vi "MP Test Path.vi"   [LabVIEW 2019]
uses:
  <vilib>/Rock Robotics/WPI/ThirdParty/Phoenix-LabVIEW/Motor Controller/Controls/CTRE_Phoenix_MotorControl_MotionProfileTrajectoryPoint.ctl
  <vilib>/Utility/file.llb/Read Delimited Spreadsheet (string).vi
  <vilib>/Rock Robotics/WPI/ThirdParty/Phoenix-LabVIEW/Motor Controller/Closed Loop/Motion Profile/CTRE_Phoenix_MotorControl_BufferedTrajectoryPointStream_WriteAll.vi
types:
  T1 = typedef "CTRE_Phoenix_MotorControl_MotionProfileTrajectoryPoint.ctl" = cluster{"Position":dbl, "Velocity":dbl, "Arbitrary Feed Forward":dbl, "Auxiliary Position":dbl, "Auxiliary Velocity":dbl, "Auxiliary Arbitrary Feed Forward":dbl, "Profile Slot Select":i32, "Auxiliary Profile Slot Select":i32, "isLastPoint?":bool, "Zero Position?":bool, "durationMs":u32, "Use Aux PID?":bool}
  T2 = typedef "CTRE_Phoenix_MotorControl_BufferedTrajectoryPointStream_DeviceRef.ctl" = cluster{"Handle":u64, "Library Path":path}
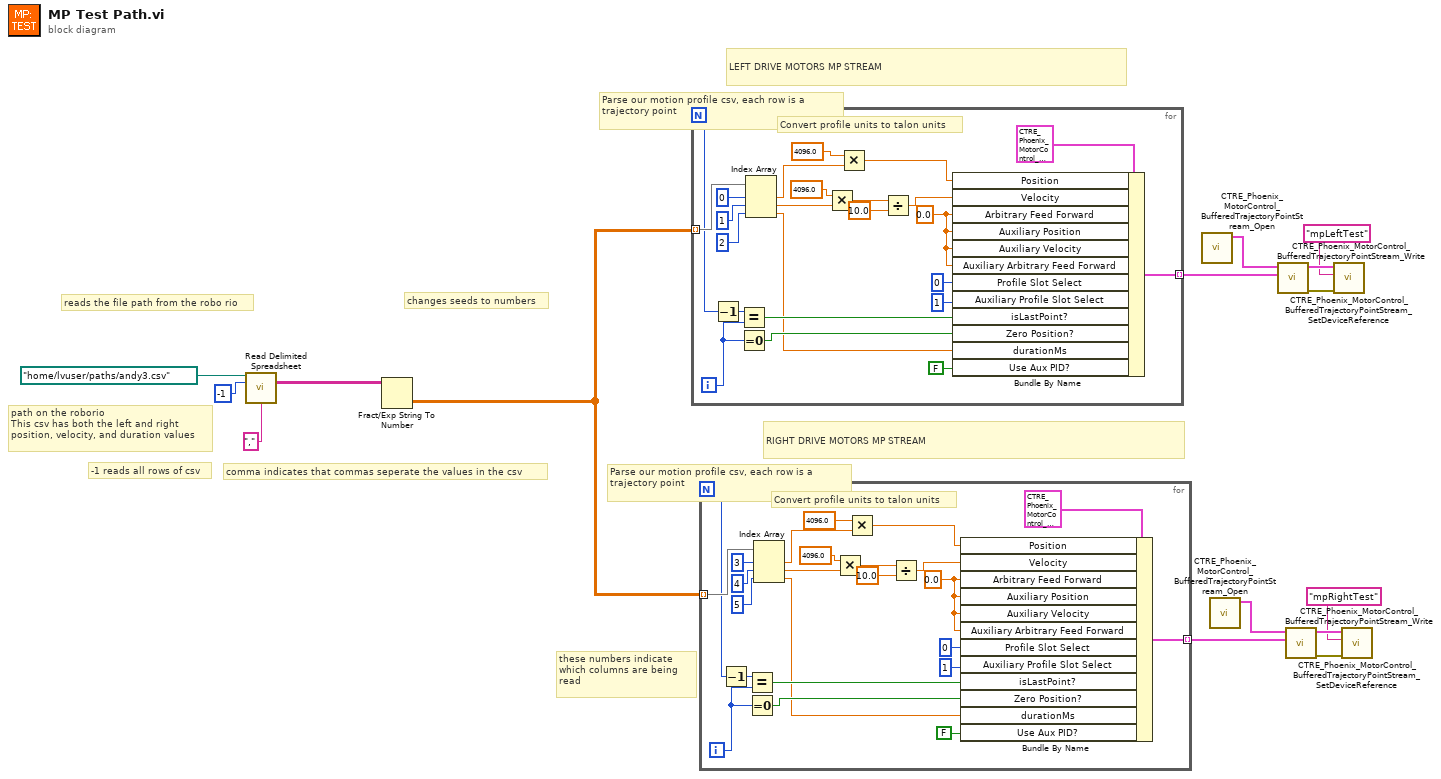
[diagram p0: block diagram]
diagram:
  # "these numbers indicate \nwhich columns are being \nread"
  # "Parse our motion profile csv, each row is a trajectory point"
  # "LEFT DRIVE MOTORS MP STREAM"
  # "Parse our motion profile csv, each row is a trajectory point"
  # "path on the roborio\nThis csv has both the left and right\nposition, velocity, and duration values"
  # "changes seeds to numbers"
  # "comma indicates that commas seperate the values in the csv"
  # "-1 reads all rows of csv"
  # "reads the file path from the robo rio"
  # "RIGHT DRIVE MOTORS MP STREAM"
  n1 = call-poly <vilib>:"Read Delimited Spreadsheet.vi"("file path (dialog if empty)"=path "/home/lvuser/paths/andy3.csv" ("file path (use dialog)"), "number of rows (all:-1)"=-1, "delimiter (\\t)"="," ("delimiter (\\t)")) -> ("all rows"=w1:string[][])  [unwired: 7 in, 5 out]
  n2 = Fract/Exp String To Number(string=w1) -> (number=w2:dbl[][])  [unwired: 3 in, 1 out]
  n3 = for {
    N -> [w32]
    tunnel: w2 -> [w38] mode=indexing
    tunnel: [w28] -> w3 mode=indexing
    i -> [w31]
    w37 = 0.0 ("Arbitrary Feed Forward")
    # "Convert profile units to talon units"
    n4 = Decrement(x=w32) -> (x-1=w33:i32)
    n5 = Equal?(x=w33, y=w31) -> (x = y?=w34:bool)
    n6 = Equal To 0?(x=w31) -> (x = 0?=w30:bool)
    n7 = Index Array(array=w38, index #1=0 ("index"), index #2=1 ("index"), index #3=2 ("index")) -> (element #1=w26:dbl, element #2=w20:dbl, element #3=w27:dbl)
    n8 = Multiply(x=4096.0, y=w20) -> (x*y=w22:dbl)
    n9 = Multiply(x=4096.0, y=w26) -> (x*y=w24:dbl)
    n10 = Divide(x=w22, y=10.0) -> (x/y=w19:dbl)
    n11 = Bundle By Name(cluster=T1 {"Position"=0.0, "Velocity"=0.0, "Arbitrary Feed Forward"=0.0, "Auxiliary Position"=0.0, "Auxiliary Velocity"=0.0, "Auxiliary Arbitrary Feed Forward"=0.0, "Profile Slot Select"=0, "Auxiliary Profile Slot Select"=0, "isLastPoint?"=FALSE, "Zero Position?"=FALSE, "durationMs"=0, "Use Aux PID?"=FALSE} ("Trajectory Point"), "Position"=w24, "Velocity"=w19, "Arbitrary Feed Forward"=w37, "Auxiliary Position"=w37, "Auxiliary Velocity"=w37, "Auxiliary Arbitrary Feed Forward"=w37, "Profile Slot Select"=0, "Auxiliary Profile Slot Select"=1, "isLastPoint?"=w34, "Zero Position?"=w30, "durationMs"=w27, "Use Aux PID?"=FALSE) -> (w28:T1)
  }
  n12 = for {
    N -> [w56]
    tunnel: w2 -> [w62] mode=indexing
    tunnel: [w52] -> w11 mode=indexing
    i -> [w55]
    w61 = 0.0 ("Arbitrary Feed Forward")
    # "Convert profile units to talon units"
    n13 = Decrement(x=w56) -> (x-1=w57:i32)
    n14 = Equal?(x=w57, y=w55) -> (x = y?=w58:bool)
    n15 = Equal To 0?(x=w55) -> (x = 0?=w54:bool)
    n16 = Index Array(array=w62, index #1=3 ("index"), index #2=4 ("index"), index #3=5 ("index")) -> (element #1=w50:dbl, element #2=w44:dbl, element #3=w51:dbl)
    n17 = Multiply(x=4096.0, y=w44) -> (x*y=w46:dbl)
    n18 = Multiply(x=4096.0, y=w50) -> (x*y=w48:dbl)
    n19 = Divide(x=w46, y=10.0) -> (x/y=w43:dbl)
    n20 = Bundle By Name(cluster=T1 {"Position"=0.0, "Velocity"=0.0, "Arbitrary Feed Forward"=0.0, "Auxiliary Position"=0.0, "Auxiliary Velocity"=0.0, "Auxiliary Arbitrary Feed Forward"=0.0, "Profile Slot Select"=0, "Auxiliary Profile Slot Select"=0, "isLastPoint?"=FALSE, "Zero Position?"=FALSE, "durationMs"=0, "Use Aux PID?"=FALSE} ("Trajectory Point"), "Position"=w48, "Velocity"=w43, "Arbitrary Feed Forward"=w61, "Auxiliary Position"=w61, "Auxiliary Velocity"=w61, "Auxiliary Arbitrary Feed Forward"=w61, "Profile Slot Select"=0, "Auxiliary Profile Slot Select"=1, "isLastPoint?"=w58, "Zero Position?"=w54, "durationMs"=w51, "Use Aux PID?"=FALSE) -> (w52:T1)
  }
  n21 = call <vilib>:"CTRE_Phoenix_MotorControl_BufferedTrajectoryPointStream_Open.vi"() -> ("BufferedTrajectoryPointStream_DevRef"=w15:T2)  [unwired: 10 in, 1 out]
  n22 = call <vilib>:"CTRE_Phoenix_MotorControl_BufferedTrajectoryPointStream_Open.vi"() -> ("BufferedTrajectoryPointStream_DevRef"=w10:T2)  [unwired: 10 in, 1 out]
  n23 = call-poly <vilib>:"CTRE_Phoenix_MotorControl_BufferedTrajectoryPointStream_Write.vi"("Motion Profile Trajectory Point Array"=w3, "BufferedTrajectoryPointStream_DevRef"=w15) -> ("error out"=w13:errorcluster, "BufferedTrajectoryPointStream_DevRef"=w14:T2)  [unwired: 8 in]
  n24 = call-poly <vilib>:"CTRE_Phoenix_MotorControl_BufferedTrajectoryPointStream_Write.vi"("Motion Profile Trajectory Point Array"=w11, "BufferedTrajectoryPointStream_DevRef"=w10) -> ("error out"=w8:errorcluster, "BufferedTrajectoryPointStream_DevRef"=w9:T2)  [unwired: 8 in]
  n25 = call <vilib>:"CTRE_Phoenix_MotorControl_BufferedTrajectoryPointStream_SetDeviceReference.vi"("error in (no error)"=w13, "refnum name"="mpLeftTest", "BufferedTrajectoryPointStream_DevRef"=w14) -> ()  [unwired: 7 in, 2 out]
  n26 = call <vilib>:"CTRE_Phoenix_MotorControl_BufferedTrajectoryPointStream_SetDeviceReference.vi"("error in (no error)"=w8, "refnum name"="mpRightTest", "BufferedTrajectoryPointStream_DevRef"=w9) -> ()  [unwired: 7 in, 2 out]
